vi "Event Handle Loop_Pop-out Panel_Release.vi"(8 "error in (no error)":errorcluster, 11 "QTab Class in":refnum<class "QTab Class.lvclass">) -> (0 "error out":errorcluster)   [LabVIEW 2020, in "QTab.lvlib" / "QTab Class.lvclass"]
uses:
  QTab Class.lvclass
  QTab Class.lvclass/QTab Class.ctl
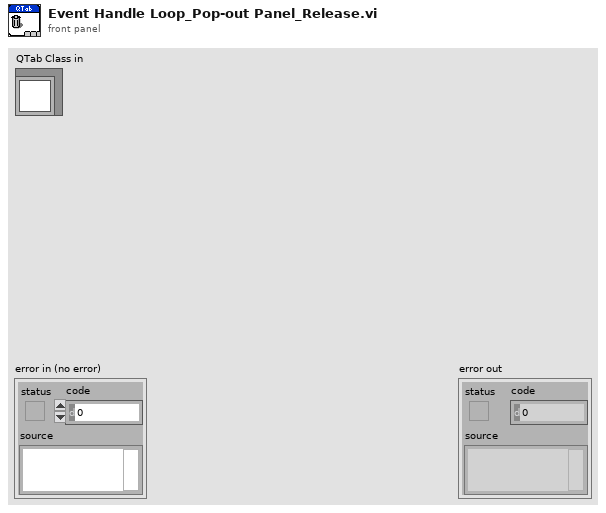
[diagram p1: front panel]
types:
  T1 = enum32{"Invalid", "Standard", "Closed", "Hidden", "Minimized", "Maximized"}
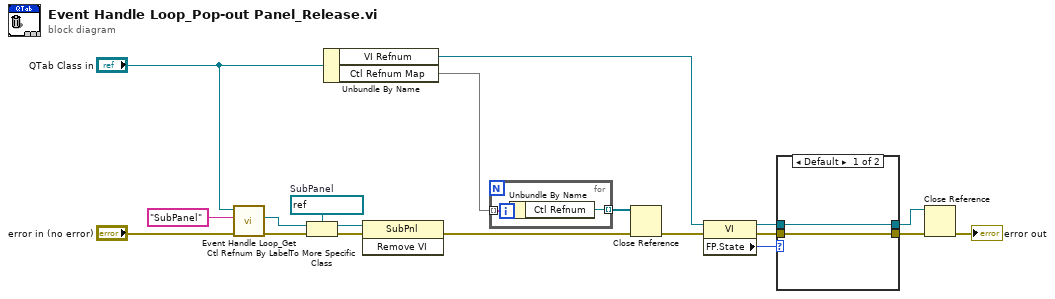
[diagram p0: block diagram]
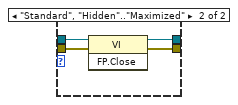
[diagram p2: hidden frame]
diagram:
  w16 = refnum<vi> refnum  # SubPanel
  n1 = call "Event Handle Loop_Get Ctl Refnum By Label.vi"("error in (no error)"="error in (no error)", "Label"="SubPanel", "QTab Class in"="QTab Class in") -> ("error out"=w18:errorcluster, "Ctl Refnum"=w17:refnum<vi>)  [unwired: 6 in, 1 out]
  n2 = To More Specific Class(target class=w16, reference=w17, error in=w18) -> (specific class reference=w14:refnum<vi>, error out=w15:errorcluster)
  n3 = Unbundle By Name("QTab Class in") -> ("VI Refnum"=w7:refnum<vi>, "Ctl Refnum Map"=w9:map{string, refnum<vi>})
  n4 = invoke class="SubPnl" method="Remove VI"(reference=w14, error in=w15) -> (error out=w10:errorcluster)  [unwired: 1 in, 2 out]
  n5 = for {
    tunnel: w9 -> [w21] mode=indexing
    tunnel: [w20] -> w11 mode=indexing
    n6 = Unbundle By Name(w21) -> ("Ctl Refnum"=w20:refnum<vi>)
  }
  n7 = Close Reference(reference=w11, error in (no error)=w10) -> (error out=w8:errorcluster)
  n8 = property class="VI"(reference=w7, error in=w8) -> (reference out=w4:refnum<vi>, error out=w5:errorcluster, "FP.State"=w6:T1)
  n9 = case shown="Default" w6 {
    tunnel: w5 -> [w22 w27]
    tunnel: w4 -> [w23 w26]
    tunnel: [w22 w25] -> w3
    tunnel: [w23 w24] -> w2
    frame Default {
    }
    frame "Standard", "Hidden".."Maximized" {
      n10 = invoke class="VI" method="FP.Close"(reference=w26, error in=w27) -> (reference out=w24:refnum<vi>, error out=w25:errorcluster)  [unwired: 1 in, 1 out]
    }
  }
  n11 = Close Reference(reference=w2, error in (no error)=w3) -> (error out=→"error out":errorcluster)
